vi "DGMM_PID_Trajectory tracking_0314.vi"() -> ()   [LabVIEW 2018]
doc: "Demonstrates the use of the Network Streams functions to send LED status to the myRIO target."
uses:
  <vilib>/addons/zeromq/socket_type.ctl
  <vilib>/ErrorRing/Error Ring.xnode
  <vilib>/vision/NI_Vision_Development_Module.lvlib
  <vilib>/addons/zeromq/zmq_context.lvclass
  <vilib>/addons/zeromq/zeromq.lvlib
  <vilib>/addons/zeromq/zmq_socket.lvclass
panel:
  in  "簇 11":T1={"next_state_x"=100000.0, "current_state_x"=1.0, "next_state_y"=100000.0, "current_state_y"=1.0}
  out "current_state_y":dbl
  out "current_state_x":dbl
  out "next_state_y":dbl
  out "next_state_x":dbl
  in  "簇 10":T2={"predicted_output_dr"=100000.0, "predicted_output_pr"=100000.0}
  in  "Operation":T3(ring)=enum."Erode"
  out "real_relative_point_y":dbl
  out "real_relative_point_x":dbl
  out "real_relative_start_point_y":dbl
  out "real_relative_start_point_x":dbl
  out "Bounding Box.Y Top 2":i32
  out "Bounding Box.X Left 2":i32
  out "Ki part":dbl
  out "Kd part":dbl
  out "Kp part":dbl
  out "Ki part":dbl
  out "Kd part":dbl
  out "Kp part":dbl
  in  "Ki":dbl=0.002
  in  "Kd":dbl=1e-05
  in  "Kp":dbl=0.005
  in  "Ki":dbl=0.002
  in  "Kd":dbl=1e-05
  in  "Kp":dbl=0.005
  out "添加的数组":dbl[](array[numeric])
  out "desired_relative_point_y":dbl=250.0
  out "desired_relative_point_x":dbl=200.0
  out "predicted_output_pr":dbl=20.0
  out "predicted_output_dr":dbl=8.0
  out "error_relative_point_y":dbl
  out "error_relative_point_x":dbl
  out "real_relative_end_point_y":dbl
  out "real_relative_end_point_x":dbl
  out "predicted_output_pr":dbl
  out "predicted_output_dr":dbl
  in  "打开仅尖端轨迹":bool
  out "仅尖端轨迹":T4(plugin-control)
  out "Bounding Box.Y Top":i32
  out "Bounding Box.X Left":i32
  out "curve_min_y":dbl
  out "curve_min_x":dbl
  out "curve_max_y":dbl
  out "curve_max_x":dbl
  out "relative_end_point_y":dbl
  out "relative_end_point_x":dbl
  out "delta_y":dbl
  out "delta_x":dbl
  out "pr":dbl
  out "tan(v)":dbl
  out "delta_velocity":dbl format="%#_10g"
  out "delta_time":dbl
  out "now time":timestamp[](array[timestamp])
  out "prev time":timestamp[](array[timestamp])
  out "delta_distance":dbl
  out "prev_end_point_y":dbl
  out "prev_end_point_x":dbl
  out "now_end_point_y":dbl
  out "now_end_point_x":dbl
  out "prev_end_point_y":dbl[](array[numeric])
  out "prev_end_point_x":dbl[](array[numeric])
  out "dr":dbl
  in  "Ar":sgl=11.0
  out "all parameters":dbl[][](array[numeric])
  out "direction angle":sgl[](array[numeric])
  out "dr":sgl
  out "strength":dbl[](array[numeric])
  out "场强":dbl
  out "end_point_y":T5
  out "end_point_x":dbl[](array[numeric])
  out "start_point_y":dbl[](array[numeric])
  out "start_point_x":dbl[](array[numeric])
  out "T":i32[](array[numeric])
  out "c":dbl[](array[numeric])
  out "b":dbl[](array[numeric])
  out "a\na":dbl[](array[numeric])
  out "c":dbl
  out "b":dbl
  out "a":dbl
  out "Angles (deg)":sgl[](array[numeric]) format="%.2f"
  in  "wr":sgl
  in  "打开轨迹":bool
  out "中心轨迹和尖端轨迹":T4(plugin-control)
  out "end_y":dbl
  out "end_x":dbl
  out "start_y":dbl
  out "start_x":dbl
  out "Image Pixels (U8)":u8[][](array[numeric])
  in  "Poly":dbl
  out "中心轨迹":T4(plugin-control)
  in  "保存按钮":bool
  out "Object Center":cluster{"X":sgl, "Y":sgl}
  out "黑白图":T4(plugin-control)
  in  "Number of Erosion":i32=5
  in  "Settings":T6={"Objects"=1, "Threshold"=128, "Reject Border"=FALSE, "Fill Holes"=FALSE, "Min Object Size"=TRUE, "Min Size"=3000, "Max Object Size"=FALSE, "Max Size"=100, "Show Search Area"=TRUE, "Show Center"=TRUE, "Show Bounding Box"=TRUE} {"Objects" items=["Bright Objects", "Dark Objects"]; "Threshold" min=1 max=999999999 step=1; "Max Size" min=1 max=999999999 step=1; "Min Size" min=1 max=999999999 step=1}
  out "Objects":T7(array[cluster]) {"Aspect Ratio" format="%.2f"; "Orientation" format="%.2f"; "Area" format="%.2f"; "Object Center"."Y" format="%.2f"; "Object Center"."X" format="%.2f"}
  in  "Search Rect (entire image)":T8={"Left"=160, "Top"=740, "Right"=1900, "Bottom"=1620, "Rotation"=0.0} {"Rotation" format="%.2f"; "Left" scale=0.0..1024.0; "Right" scale=0.0..1024.0}
  in  "Range":cluster{"Lower value":sgl, "Upper value":sgl}={"Lower value"=181.0, "Upper value"=255.0} {"Upper value" format="%.2f"; "Lower value" format="%.2f"}
  out "原图":T4(plugin-control)
  in  "停止":bool
  out "T":i32
  out "T":i32
  in  "磁场变换":bool=TRUE
  in  "Pause":bool
  out "Array":ext[](array[numeric])
  in  "Parameter Settings":T9(tab)=enum."Rotating Field" caption="Field Types"
  in  "Ag":dbl
  in  "dg":dbl
  in  "pg":dbl
  in  "fg":dbl
  in  "AoOF":dbl
  in  "fo":sgl
  in  "do":sgl
  in  "oo":sgl
  in  "po":sgl
  in  "cc":sgl
  in  "pc":sgl
  in  "wc":sgl
  in  "dc":sgl
  in  "Ac":dbl
  in  "Dis phase step":dbl
  in  "Dis phase frequency (Hz)":dbl
  in  "Dis tumbling frequency (Hz)":dbl
  in  "Dis strength(mT)":dbl
  in  "Swa strength (mT)":dbl
  in  "Swa frequency (Hz)":dbl
  in  "Swa pitch angle (deg)":dbl
  in  "Swa direction angle (deg)":dbl
  in  "Swa ratio":dbl=1.0
  in  "Pitch Angle (rotating around Constant, deg)":dbl
  in  "Ratio (A/C)":sgl
  in  "Direction Angle (deg)":sgl
  in  "Pitch Angle (rotating around Origin, deg)":sgl
  in  "Frequency (Hz)":sgl
  in  "Strength (mT)":dbl
  in  "Ar 2":dbl caption="Ar"
  in  "ratio":sgl
  in  "pr  2":sgl
  in  "dr  2":sgl
  in  "wr  2":sgl
  in  "p_x":sgl
  out "Numeric 5":i32
  in  "Stop":bool
  out "error out":errorcluster
  in  "Target IP Address":string="172.22.11.2"
  # "Overview: Magnetic field calculation, and send parameters to myRIO\nInstructions:\n1. Verify the value of Target IP Address. Set Visa resource name.\n2. Ensure RT Main.vi is already running. \n3. Run this VI. Set parameters of magnetic field."
  # "Strength (mT)"
  # "Frequency (Hz)"
  # "Pitch Angle (deg)"
  # "Direction Angle (deg)"
  # "Strength (mT)"
  # "Pitch Angle (deg)"
  # "Direction Angle (deg)"
  # "Frequency (Hz)"
  # "Strength (mT)"
  # "Oscilation Frequency (Hz)"
  # "Oscilation Angle (deg)"
  # "Pitch Angle (deg)"
  # "Direction Angle (deg)"
  # "Strength (mT)"
  # "Frequency (Hz)"
  # "Pitch Angle (deg)"
  # "Direction Angle (deg)"
  # "Conical Angle (deg)"
  # "Strength (mT)"
  # "Tumbling Frequency (Hz)"
  # "Phase Frequency (Hz)"
  # "Phase Step"
  # "Strength (mT)"
  # "Frequency (Hz)"
  # "Pitch Angle (deg)"
  # "Direction Angle (deg)"
  # "Ratio"
  # "Strength (mT)"
  # "Frequency (Hz)"
  # "Ratio (A/C)"
  # "Direction Angle (deg)"
  # "Pitch Angle (rotating around Origin, deg)"
  # "Pitch Angle (rotating around Constant, deg)"
  # "Strength (mT)"
  # "Frequency (Hz)"
  # "Pitch Angle Y (deg)"
  # "Pitch Angle X (deg)"
  # "Direction Angle (deg)"
  # "ratio (l/s)"
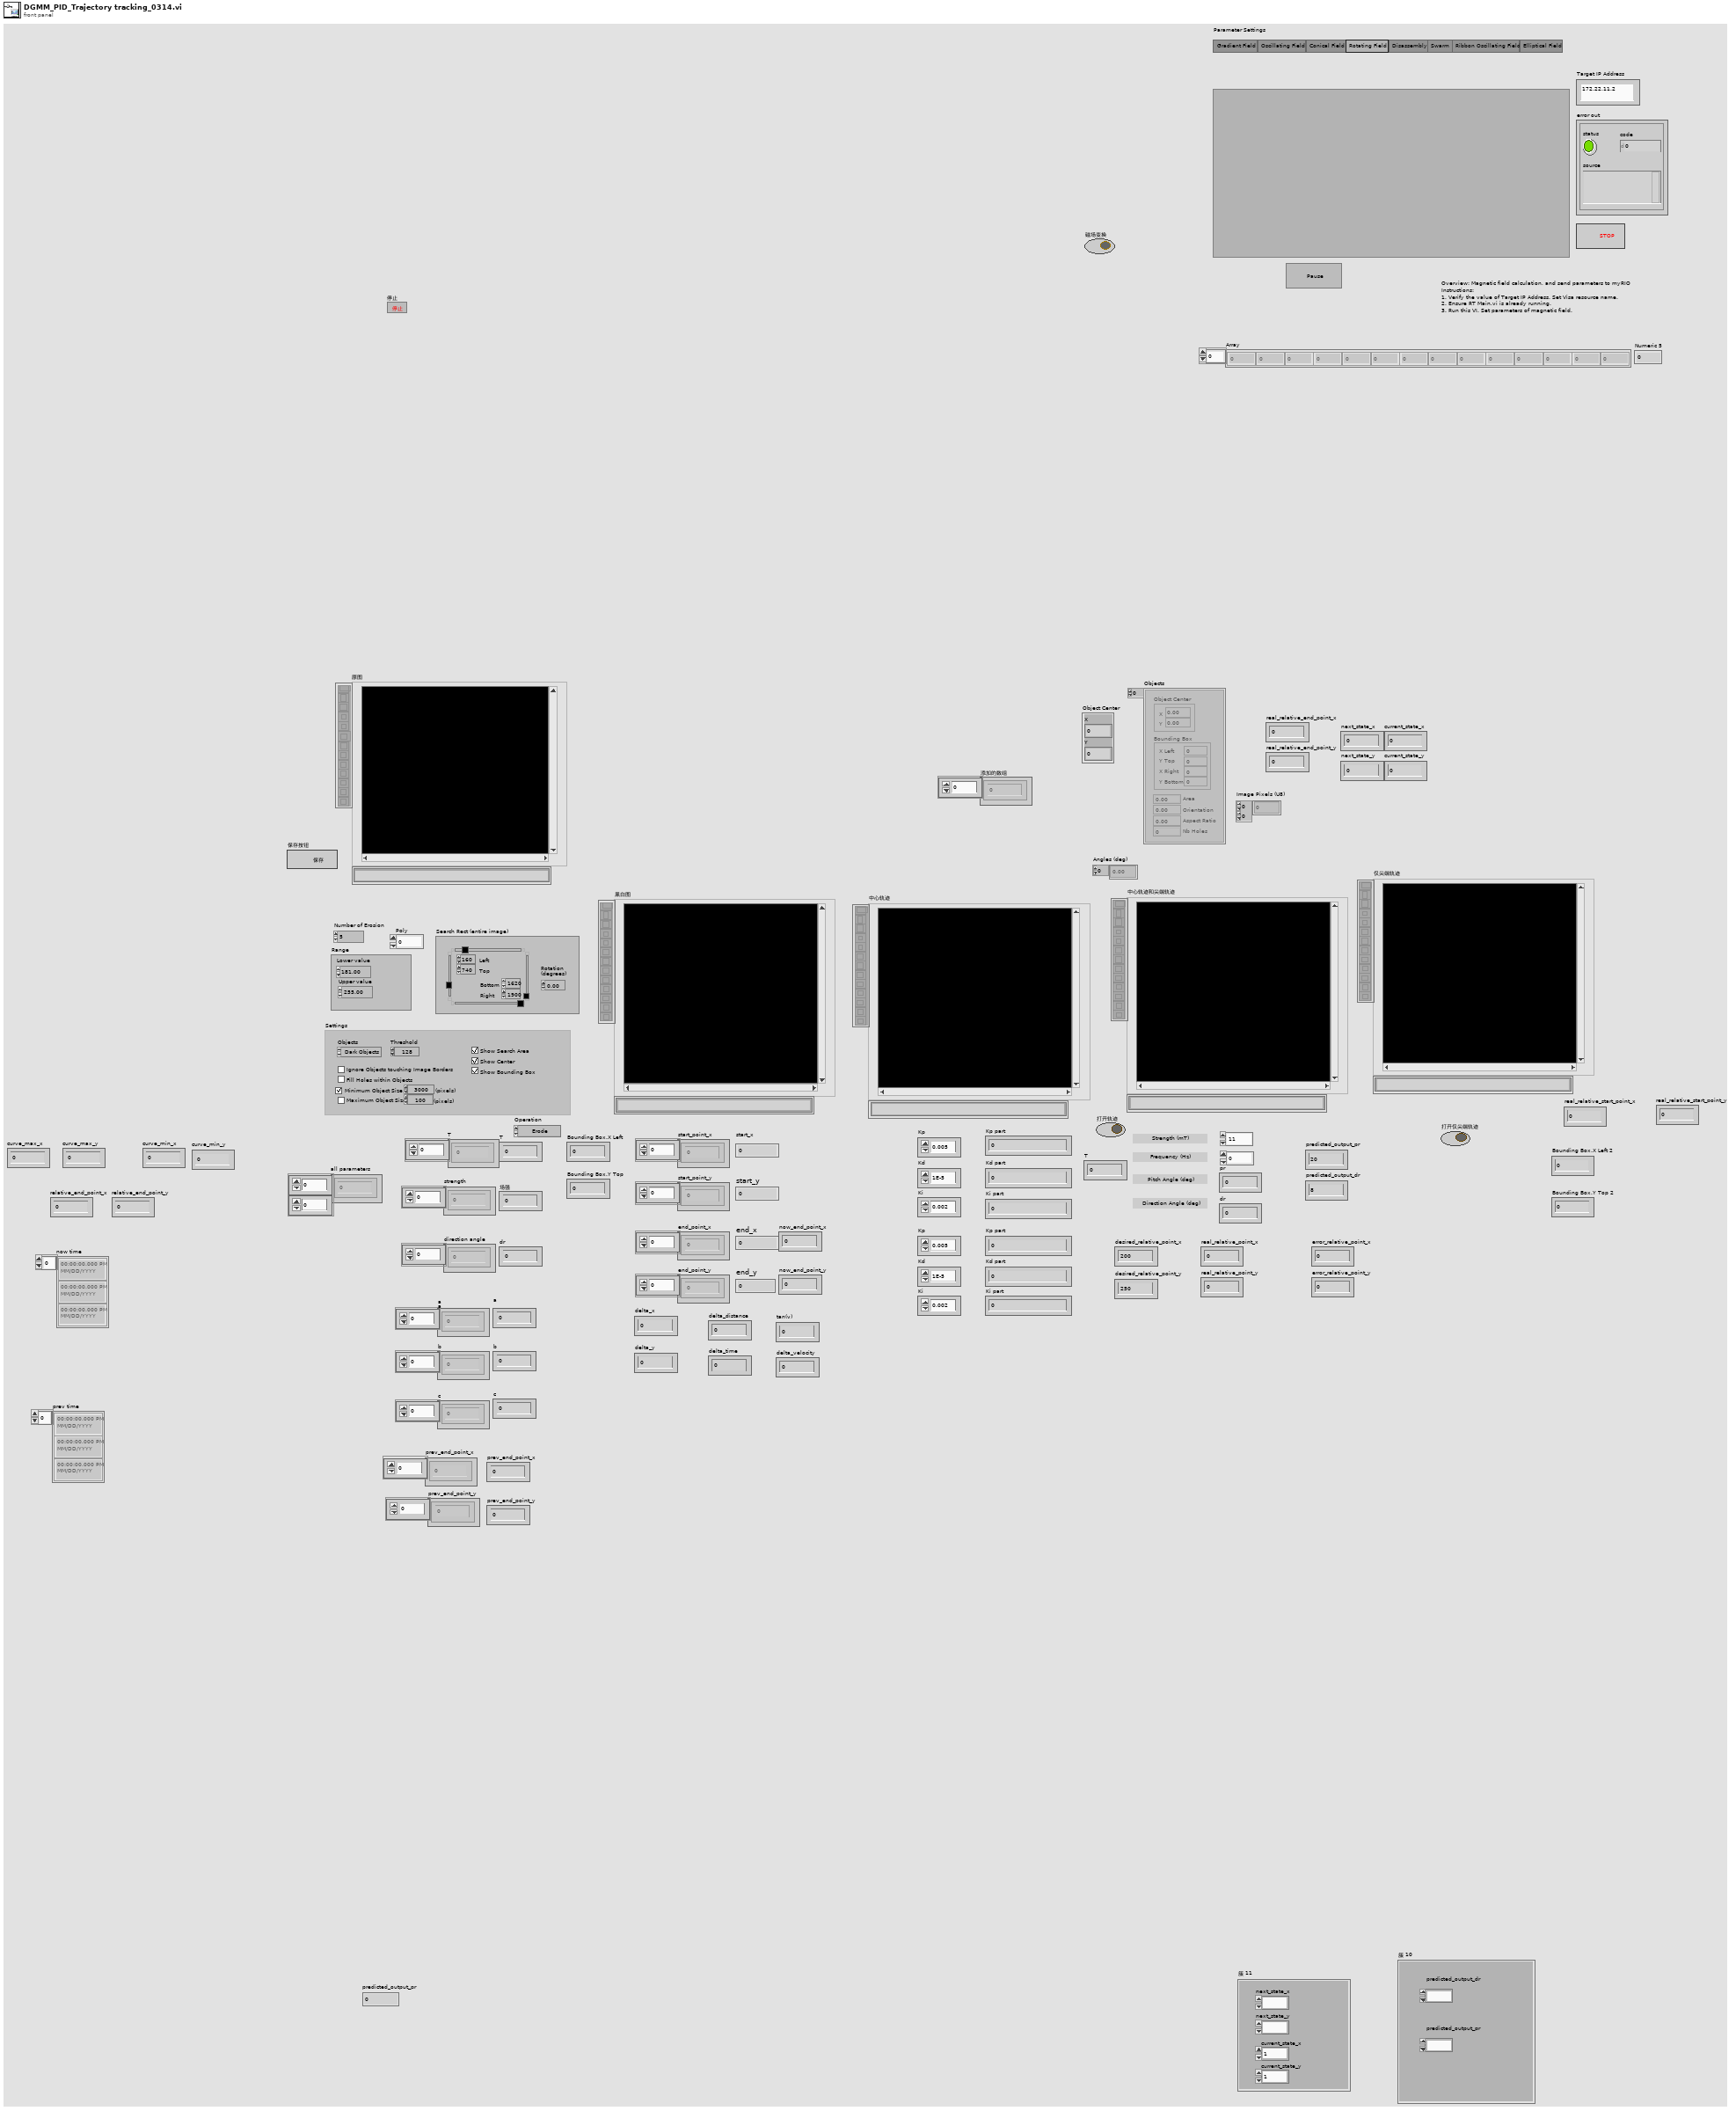
[diagram p1: front panel]
types:
  T1 = cluster{"next_state_x":ext, "current_state_x":dbl, "next_state_y":ext, "current_state_y":dbl}
  T2 = cluster{"predicted_output_dr":ext, "predicted_output_pr":ext}
  T3 = enum32{"AutoM", "Close", "Dilate", "Erode", "Gradient", "Gradient in", "Gradient out", "HitMiss", "Open", "PClose", "POpen", "Thick", "Thin"}
  T4 = typedef "IMAQ Image.ctl" = refnum<image>
  T5 = typedef "控件 3.ctl" = dbl[]
  T6 = cluster{"Objects":u16, "Threshold":i32, "Reject Border":bool, "Fill Holes":bool, "Min Object Size":bool, "Min Size":i32, "Max Object Size":bool, "Max Size":i32, "Show Search Area":bool, "Show Center":bool, "Show Bounding Box":bool}
  T7 = cluster{"Object Center":cluster{"X":sgl, "Y":sgl}, "Bounding Box":cluster{"X Left":i32, "Y Top":i32, "X Right":i32, "Y Bottom":i32}, "Area":sgl, "Orientation":sgl, "Aspect Ratio":sgl, "Nb Holes":i32}[]
  T8 = typedef "IMAQ Rectangle" = cluster{"Left":i32, "Top":i32, "Right":i32, "Bottom":i32, "Rotation":dbl}
  T9 = enum32{"Gradient Field ", "Oscillating Field", "Conical Field", "Rotating Field", "Disassembly", "Swarm", "Ribbon Oscillating Field", "Elliptical Field"}
  T10 = typedef "zeromq.lvlib/socket_type.ctl" = enum8{"ZMQ_PAIR", "ZMQ_PUB", "ZMQ_SUB", "ZMQ_REQ", "ZMQ_REP", "ZMQ_DEALER", "ZMQ_ROUTER", "ZMQ_PULL", "ZMQ_PUSH", "ZMQ_XPUB", "ZMQ_XSUB", "ZMQ_STREAM", "ZMQ_SERVER", "ZMQ_CLIENT", "ZMQ_RADIO", "ZMQ_DISH", "ZMQ_GATHER", "ZMQ_SCATTER", "ZMQ_DGRAM"}
  T11 = typedef "Image Type" = u32
  T12 = cluster{"Object Center":cluster{"X":sgl, "Y":sgl}, "Bounding Box":cluster{"X Left":i32, "Y Top":i32, "X Right":i32, "Y Bottom":i32}, "Area":sgl, "Orientation":sgl, "Aspect Ratio":sgl, "Nb Holes":i32}
  T13 = cluster{"X Left":i32, "Y Top":i32, "X Right":i32, "Y Bottom":i32, "Rotation":dbl}
  T14 = typedef "ROI Descriptor" = cluster{"Global Rectangle":i32[], "Contours":cluster{"ID":enum32{"External", "Internal"}, "Type":u32, "Coordinates":i32[]}[]}
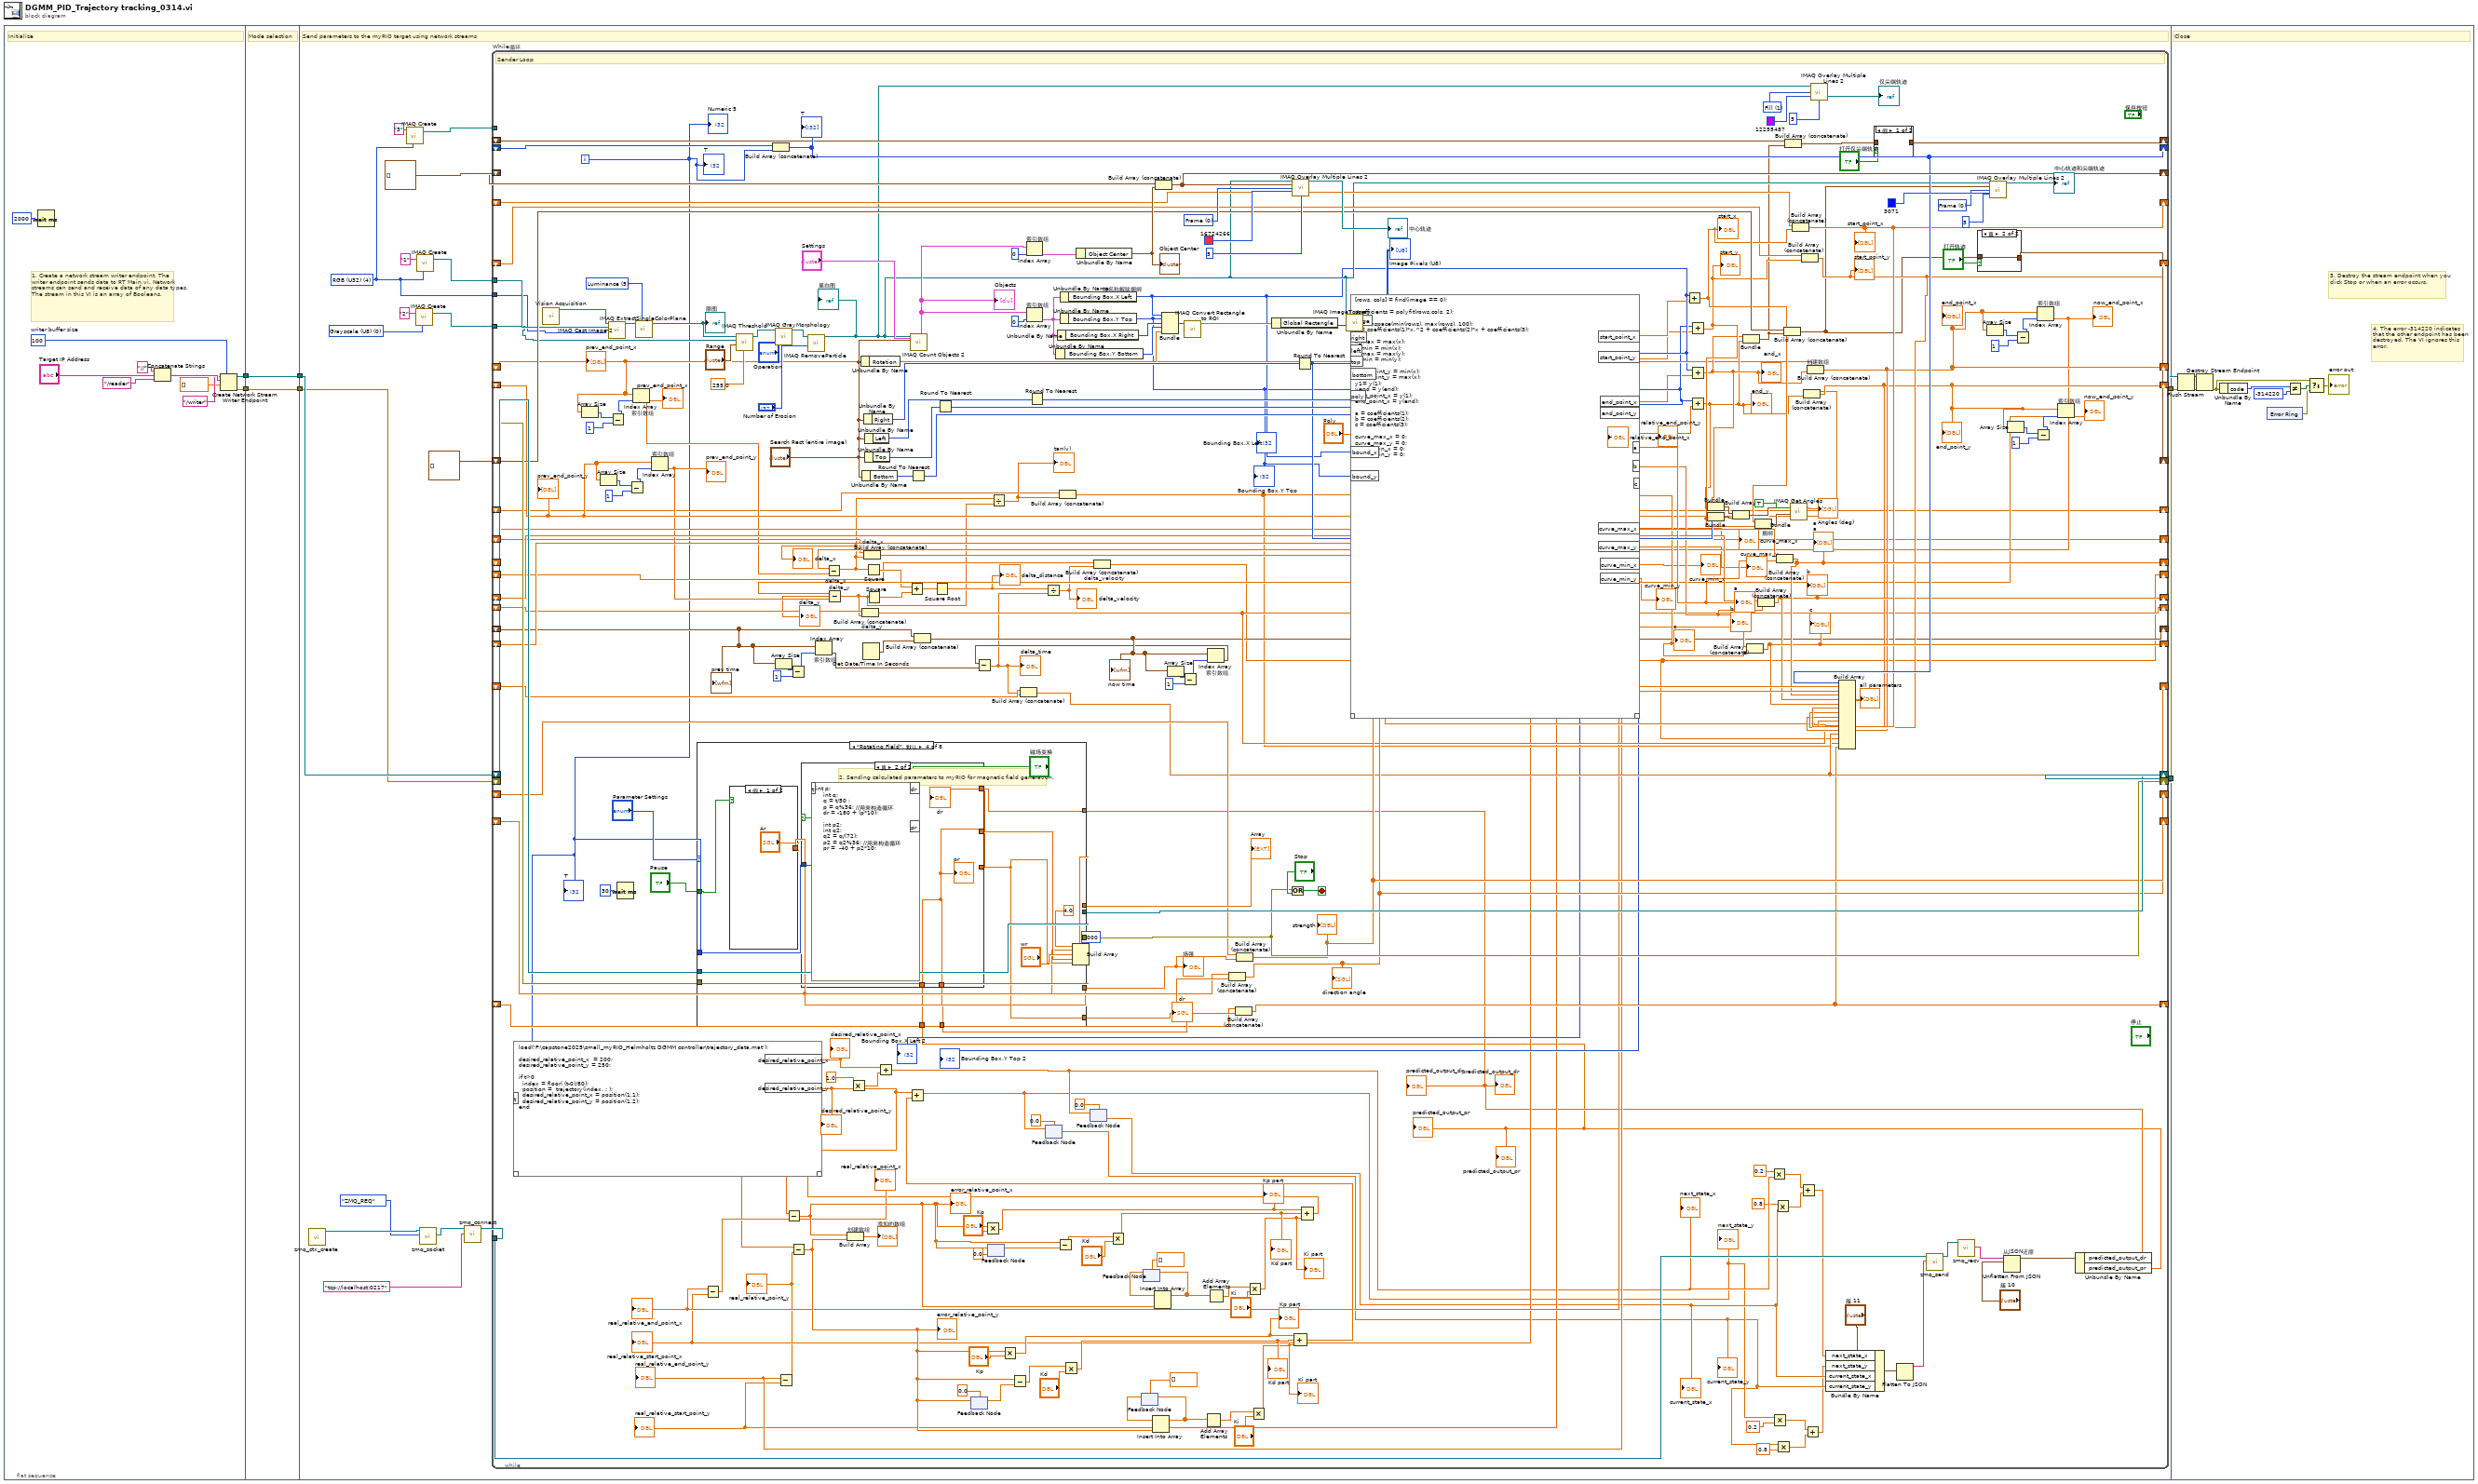
[diagram p0: block diagram]
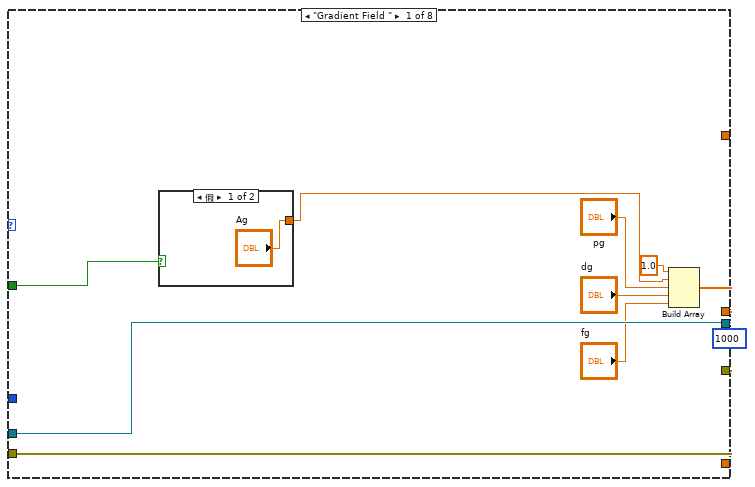
[diagram p4: hidden frame]
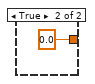
[diagram p5: hidden frame]
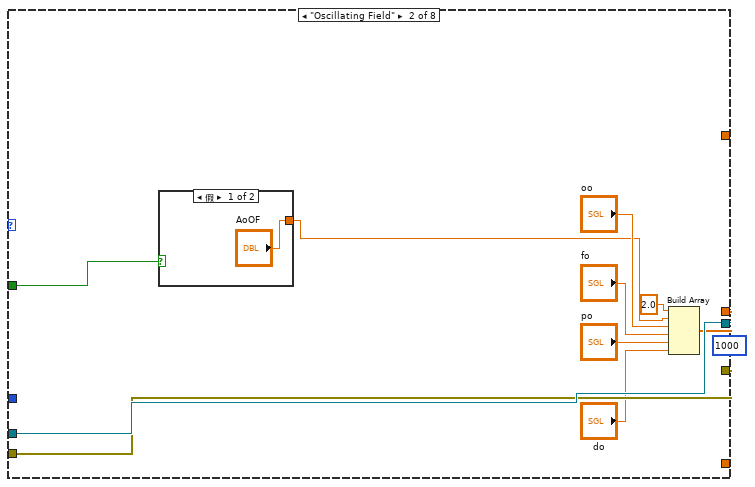
[diagram p6: hidden frame]
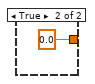
[diagram p7: hidden frame]
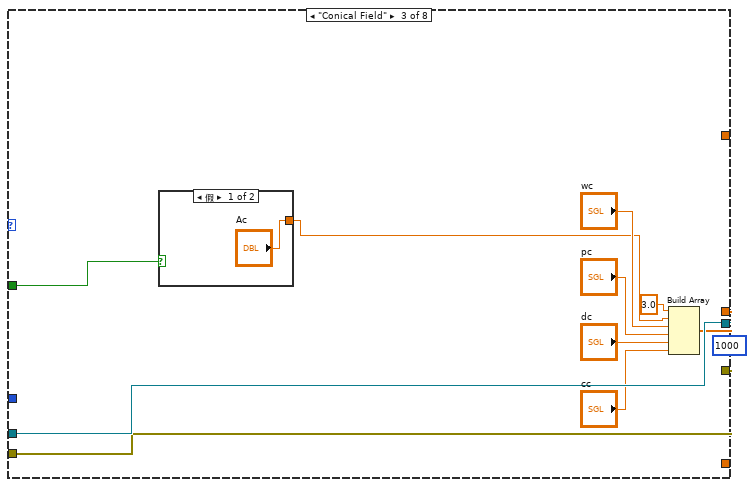
[diagram p8: hidden frame]
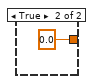
[diagram p9: hidden frame]
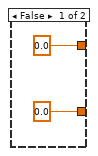
[diagram p10: hidden frame]
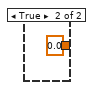
[diagram p11: hidden frame]
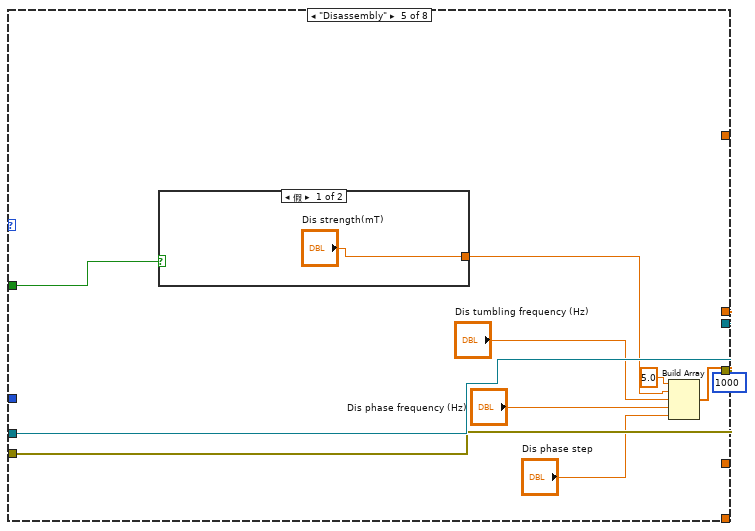
[diagram p12: hidden frame]
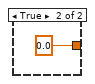
[diagram p13: hidden frame]
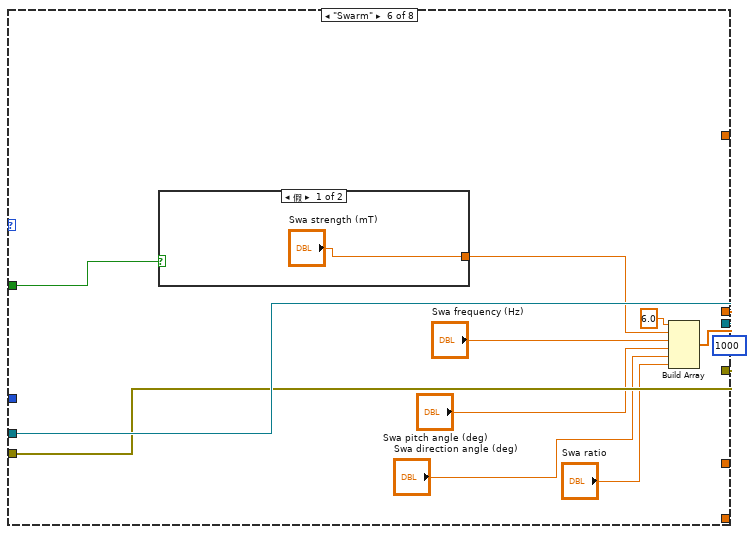
[diagram p14: hidden frame]
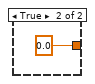
[diagram p15: hidden frame]
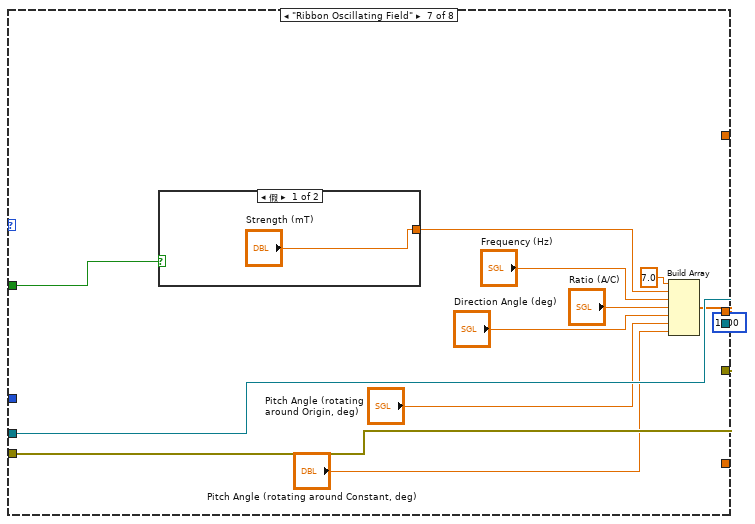
[diagram p16: hidden frame]
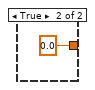
[diagram p17: hidden frame]
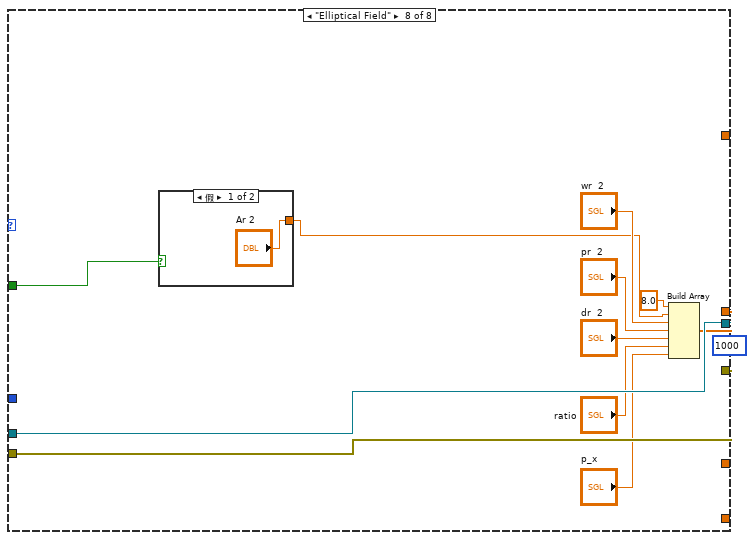
[diagram p18: hidden frame]
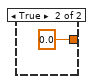
[diagram p19: hidden frame]
diagram:
  n1 = flat-sequence {
    tunnel: [w11] -> w2
    tunnel: [w10] -> w1
    tunnel: [w18] -> w4
    tunnel: [w17] -> w3
    tunnel: w1 -> [w17]
    tunnel: w2 -> [w18]
    tunnel: [w35] -> w6
    tunnel: w4 -> [w37]
    tunnel: [w34] -> w5
    tunnel: w3 -> [w36]
    tunnel: w6 -> [w408]
    tunnel: w5 -> [w405]
    frame #0 {
      w9 = 100  # writer buffer size
      # "1. Create a network stream writer endpoint. The writer endpoint sends data to RT Main.vi. Network streams can send and receive data of any data types. The stream in this VI is an array of Booleans."
      # "Initialize"
      n2 = Wait (ms)(milliseconds to wait=2000) -> ()  [unwired: 1 out]
      n3 = Concatenate Strings("//", "Target IP Address", "/reader") -> (w16:string)
      n4 = Create Network Stream Writer Endpoint(7:w9, 9:dbl[] [], 10:w16, 11:"/writer" ("reader name")) -> (0:w10:errorcluster, 3:w11:refnum<k21>)  [unwired: 3 in]
    }
    frame #1 {
      # "Mode selection"
    }
    frame #2 {
      w31 = T11 0 items=["Grayscale (U8)", "Grayscale (I16)", "Grayscale (SGL)", "Complex (CSG)", "RGB (U32)", "HSL (U32)", "RGB (U64)", "Grayscale (U16)"] ("Image Type")
      w24 = T11 4 items=["Grayscale (U8)", "Grayscale (I16)", "Grayscale (SGL)", "Complex (CSG)", "RGB (U32)", "HSL (U32)", "RGB (U64)", "Grayscale (U16)"] ("Image Type")
      # "Send parameters to the myRIO target using network streams"
      n5 = call <vilib>:"zmq_ctx_create.vi"() -> ("context out"=w22:refnum<class "zmq_context.lvclass">)  [unwired: 4 in, 1 out]
      n6 = call "IMAQ Create"("Image Name"="3", "Image Type"=w24) -> ("New Image"=w27:T4)  [unwired: 3 in, 1 out]
      n7 = call "IMAQ Create"("Image Name"="2", "Image Type"=w31) -> ("New Image"=w29:T4)  [unwired: 3 in, 1 out]
      n8 = call "IMAQ Create"("Image Name"="1", "Image Type"=w24) -> ("New Image"=w30:T4)  [unwired: 3 in, 1 out]
      n9 = call <vilib>:"zmq_socket.vi"("socket type"=socket_type."ZMQ_REQ", "context in"=w22) -> ("socket out"=w23:refnum<class "zmq_socket.lvclass">)  [unwired: 3 in, 2 out]
      n10 = call <vilib>:"zmq_connect.vi"("endpoint"="tcp://localhost:0217", "socket in"=w23) -> ("socket out"=w19:refnum<class "zmq_socket.lvclass">)  [unwired: 2 in, 1 out]
      n11 = while "While循环" {
        shift-right: [w263] -> w34
        shift-left: w36 -> [w265]
        shift-right: [w264] -> w35
        shift-left: w37 -> [w266]
        tunnel: w30 -> [w217]
        tunnel: w29 -> [w216]
        tunnel: w27 -> [_]
        shift-right: [w213] -> _
        shift-left: cluster{"X":dbl, "Y":dbl}[] [] -> [w218]
        shift-right: [w219] -> _
        shift-left: cluster{"X":dbl, "Y":dbl}[] [] -> [w220]
        tunnel: w24 -> [w215]
        shift-right: [w185] -> _
        shift-left: _ -> [w205]
        shift-right: [w180] -> _
        shift-left: _ -> [w203]
        shift-right: [w184] -> _
        shift-left: _ -> [w200]
        shift-right: [w188] -> _
        shift-left: _ -> [w199]
        shift-right: [w183] -> _
        shift-left: _ -> [w197]
        shift-right: [w182] -> _
        shift-left: _ -> [w195]
        shift-right: [w176] -> _
        shift-left: _ -> [w168]
        shift-right: [w172] -> _
        shift-left: _ -> [w164]
        shift-right: [w187] -> _
        shift-left: _ -> [w191]
        shift-right: [w186] -> _
        shift-left: _ -> [w189]
        shift-right: [w153] -> _
        shift-left: _ -> [w155]
        shift-right: [w152] -> _
        shift-left: _ -> [w154]
        shift-right: [w142] -> _
        shift-left: _ -> [w147]
        shift-right: [w139] -> _
        shift-left: _ -> [w140]
        shift-right: [w135] -> _
        shift-left: _ -> [w136]
        shift-right: [w130] -> _
        shift-left: _ -> [w131]
        shift-right: [w122] -> _
        shift-left: _ -> [w123]
        shift-right: [w116] -> _
        shift-left: _ -> [w117]
        tunnel: w19 -> [w56]
        i -> [w110]
        stop <- w259 stop-if-true
        w118 = u32 1 items=["Frame", "Fill"] ("Drawing Mode (Frame)")
        w125 = u32 0 items=["Frame", "Fill"] ("Drawing Mode (Frame)")
        w246 = u32 0 items=["Frame", "Fill"] ("Drawing Mode (Frame)")
        w256 = 5 items=["Red", "Green", "Blue", "Hue", "Saturation", "Luminance", "Value", "Intensity"] ("Color Plane")
        # "2. Sending calculated parameters to myRIO for magnetic field generation."
        # "Sender Loop"
        n12 = script code="load('F:\\capstone2025\\small_myRIO_Helmholtz DGMM controller\\trajectory_data.mat');\n\ndesired_relative_point_x  = 200;\ndesired_relative_point_y = 250;\n\nif t>0\n  index = floor( (t-0)/80); \n  position =  trajectory(index, : );\n  desired_relative_point_x = position(1,1);\n  desired_relative_point_y = position(1,2);\nend"("t"=w110) -> ("desired_relative_point_x"=w64:dbl, "desired_relative_point_y"=w65:dbl)  [unwired: 1 in, 1 out]
        "desired_relative_point_x" <- w64
        "desired_relative_point_y" <- w65
        n13 = call "Vision Acquisition"() -> ("Image Out"=w244:T4)  [unwired: 23 in, 4 out]
        n14 = Array Size(array=w168) -> (size(s)=w170:i32)
        n15 = Array Size(array=w164) -> (size(s)=w166:i32)
        n16 = call "IMAQ Cast Image 2"("Image Src"=w244, "Image Dst"=w217, "Image Type"=w215) -> ("Image Dst Out"=w257:T4)  [unwired: 11 in, 1 out]
        n17 = Subtract(x=w170, y=1) -> (x-y=w169:i32)
        n18 = Wait (ms)(milliseconds to wait=u32 30 ("等待时间（毫秒）")) -> ()  [unwired: 1 out]
        n19 = Subtract(x=w166, y=1) -> (x-y=w165:i32)
        n20 = Index Array "索引数组"(array=w168, index=w169) -> (element=w162:dbl)
        "prev_end_point_x" <- w162
        n21 = call "IMAQ ExtractSingleColorPlane"("Color Plane"=w256, "Image Src"=w257) -> ("Image Dst Out"=w255:T4)  [unwired: 8 in, 1 out]
        "原图" <- w255
        n22 = Index Array "索引数组"(array=w164, index=w165) -> (element=w161:dbl)
        "prev_end_point_y" <- w161
        n23 = call "IMAQ Threshold"("Replace Value"=sgl 255.0, "Range"="Range", "Image Dst"=w216, "Image Src"=w255) -> ("Image Dst Out"=w71:T4)  [unwired: 6 in, 1 out]
        n24 = Build Array (concatenate)(w199, w110) -> (w188:i32[])
        "T" <- w188
        n25 = call "IMAQ GrayMorphology"("Operation"="Operation", "Image Src"=w71) -> ("Image Dst Out"=w70:T4)  [unwired: 8 in, 1 out]
        n26 = Array Size(array=w147) -> (size(s)=w150:i32)
        n27 = Subtract(x=w150, y=1) -> (x-y=w149:i32)
        n28 = call "IMAQ RemoveParticle"("Number of Erosion"="Number of Erosion", "Image Src"=w70) -> ("Image Dst Out"=w114:T4)  [unwired: 8 in, 1 out]
        "黑白图" <- w114
        n29 = Index Array "索引数组"(array=w147, index=w149) -> (element=w146:timestamp)
        n30 = Unbundle By Name("Search Rect (entire image)") -> ("Rotation"=w241:dbl)
        n31 = Unbundle By Name("Search Rect (entire image)") -> ("Bottom"=w225:i32)
        n32 = Get Date/Time In Seconds() -> (seconds since 1Jan1904=w151:timestamp)
        n33 = Unbundle By Name("Search Rect (entire image)") -> ("Right"=w229:i32)
        n34 = Unbundle By Name("Search Rect (entire image)") -> ("Left"=w228:i32)
        n35 = Unbundle By Name("Search Rect (entire image)") -> ("Top"=w227:i32)
        n36 = Round To Nearest(number=w225) -> (nearest integer value=w224:i32)
        n37 = call "IMAQ Count Objects 2"("Settings"="Settings", "Search Rect (entire image)"="Search Rect (entire image)", "Image"=w114) -> ("Objects"=w243:T7)  [unwired: 4 in, 4 out]
        "Objects" <- w243
        n38 = Build Array (concatenate)(w147, w151) -> (w142:timestamp[])
        "now time" <- w142
        n39 = Round To Nearest(number=w227) -> (nearest integer value=w226:i32)
        n40 = feedback #1(0.0) -> (w92:dbl)
        n41 = feedback #2(0.0) -> (w106:dbl)
        n42 = Index Array "索引数组"(array=w243, index=0 ("索引")) -> (element=w249:T12)
        n43 = Index Array "索引数组"(array=w243, index=0 ("索引")) -> (element=w239:T12)
        n44 = Round To Nearest(number=w228) -> (nearest integer value=w222:i32)
        n45 = feedback #3(0.0) -> (w42:dbl)
        "current_state_y" <- w42
        n46 = Unbundle By Name(w239) -> ("Bounding Box.Y Bottom"=w233:i32)
        n47 = Unbundle By Name(w239) -> ("Bounding Box.X Right"=w234:i32)
        n48 = Unbundle By Name "按名称解除捆绑"(w239) -> ("Bounding Box.X Left"=w79:i32)
        "Bounding Box.X Left" <- w79
        "Bounding Box.X Left 2" <- w79
        n49 = Unbundle By Name(w239) -> ("Bounding Box.Y Top"=w78:i32)
        "Bounding Box.Y Top" <- w78
        "Bounding Box.Y Top 2" <- w78
        n50 = Unbundle By Name(w249) -> ("Object Center"=w248:cluster{"X":sgl, "Y":sgl})
        "Object Center" <- w248
        n51 = feedback #4(0.0) -> (w49:dbl)
        "current_state_x" <- w49
        n52 = feedback #5(dbl[] []) -> (w87:dbl[])
        n53 = feedback #6(dbl[] []) -> (w101:dbl[])
        n54 = Build Array (concatenate)(w220, w248) -> (w219:cluster{"X":dbl, "Y":dbl}[])
        n55 = Bundle("X Left"=w79, "Y Top"=w78, "X Right"=w234, "Y Bottom"=w233, "Rotation"=w241) -> (w240:T13)  [unwired: 1 in]
        n56 = Array Size(array=w142) -> (size(s)=w145:i32)
        n57 = Subtract(x=w145, y=1) -> (x-y=w144:i32)
        n58 = call "IMAQ Convert Rectangle to ROI"("Rectangle"=w240) -> ("ROI Descriptor"=w238:T14)  [unwired: 8 in, 1 out]
        n59 = Index Array "索引数组"(array=w142, index=w144) -> (element=w141:timestamp)
        n60 = Subtract(x=w141, y=w146) -> (x-y=w138:dbl)
        "delta_time" <- w138
        n61 = Build Array (concatenate)(w140, w138) -> (w139:dbl[])
        n62 = Unbundle By Name(w238) -> ("Global Rectangle"=w223:i32[])
        n63 = call "IMAQ Overlay Multiple Lines 2"("Image"=w114, "Line End Points"=w219, "Drawing Mode (Frame)"=w246, "Color"=u32 16724266, "Width"=u32 5) -> ("Image Out"=→"中心轨迹":T4)  [unwired: 9 in, 1 out]
        n64 = Round To Nearest(number=w229) -> (nearest integer value=w206:i32)
        n65 = call "IMAQ ImageToArray"("Optional Rectangle"=w223, "Image"=w114) -> ("Image Pixels (U8)"=w235:u8[][])  [unwired: 2 in, 4 out]
        "Image Pixels (U8)" <- w235
        n66 = script code="[rows, cols] = find(image == 0); \n\ncoefficients = polyfit(rows,cols, 2);\n\nx = linspace(min(rows), max(rows), 100); \ny = coefficients(1)*x.^2 + coefficients(2)*x + coefficients(3);\n\nx_max = max(x);\nx_min = min(x);\ny_max = max(y);\ny_min = min(y);\n\nstart_point_y = min(x);\nend_point_y = max(x);\ny1= y(1);\nyend = y(end);\nstart_point_x = y(1);\nend_point_x = y(end);\n\na = coefficients(1);\nb = coefficients(2);\nc = coefficients(3);\n\ncurve_max_x = 0;\ncurve_max_y = 0;\ncurve_min_x = 0;\ncurve_min_y = 0;"("image"=w235, "poly"="Poly", "right"=w206, "left"=w222, "top"=w226, "bottom"=w224, "bound_x"=w79, "bound_y"=w78) -> ("start_point_x"=w76:dbl, "start_point_y"=w73:dbl, "end_point_x"=w77:dbl, "end_point_y"=w74:dbl, "a"=w204:dbl, "b"=w202:dbl, "c"=w201:dbl, "curve_max_x"=→"curve_max_x":dbl, "curve_max_y"=→"curve_max_y":dbl, "curve_min_x"=→"curve_min_x":dbl, "curve_min_y"=→"curve_min_y":dbl)  [unwired: 1 in, 1 out]
        "a" <- w204
        "b" <- w202
        "c" <- w201
        "relative_end_point_x" <- w77
        "relative_end_point_y" <- w74
        "real_relative_end_point_x" <- w77
        "real_relative_end_point_y" <- w74
        "real_relative_start_point_x" <- w76
        "real_relative_start_point_y" <- w73
        n67 = Subtract(x=w77, y=w76) -> (x-y=w75:dbl)
        "real_relative_point_x" <- w75
        n68 = Subtract(x=w74, y=w73) -> (x-y=w72:dbl)
        "real_relative_point_y" <- w72
        n69 = Subtract(x=w64, y=w75) -> (x-y=w100:dbl)
        "error_relative_point_x" <- w100
        n70 = Subtract(x=w65, y=w72) -> (x-y=w85:dbl)
        "error_relative_point_y" <- w85
        n71 = Build Array "创建数组"(w100, w85) -> (→"添加的数组":dbl[])
        n72 = feedback-in #1(w85) -> ()
        n73 = Multiply(x=w100, y="Kp") -> (x*y=w107:dbl)
        "Kp part" <- w107
        n74 = feedback-in #2(w100) -> ()
        n75 = Multiply(x=w85, y="Kp") -> (x*y=w93:dbl)
        "Kp part" <- w93
        n76 = Subtract(x=w85, y=w92) -> (x-y=w90:dbl)
        n77 = Subtract(x=w100, y=w106) -> (x-y=w104:dbl)
        n78 = Multiply(x=w90, y="Kd") -> (x*y=w88:dbl)
        "Kd part" <- w88
        n79 = Multiply(x=w104, y="Kd") -> (x*y=w102:dbl)
        "Kd part" <- w102
        n80 = Insert Into Array(array=w87, new element=w85) -> (w86:dbl[])  [unwired: 1 in]
        n81 = feedback-in #5(w86) -> ()
        n82 = Insert Into Array(array=w101, new element=w100) -> (w99:dbl[])  [unwired: 1 in]
        n83 = feedback-in #6(w99) -> ()
        n84 = Add Array Elements(numeric array=w86) -> (sum=w83:dbl)
        n85 = Add Array Elements(numeric array=w99) -> (sum=w97:dbl)
        n86 = Multiply(x=w97, y="Ki") -> (x*y=w95:dbl)
        "Ki part" <- w95
        n87 = Multiply(x=w83, y="Ki") -> (x*y=w81:dbl)
        "Ki part" <- w81
        n88 = Compound Arithmetic op=ADD(w93, w88, w81) -> (w80:dbl)
        n89 = Add(x=w65, y=w80) -> (x+y=w44:dbl)
        "next_state_y" <- w44
        n90 = feedback-in #3(w44) -> ()
        n91 = Compound Arithmetic op=ADD(w107, w102, w95) -> (w68:dbl)
        n92 = Multiply(x=1.0, y=w68) -> (x*y=w66:dbl)
        n93 = Add(x=w64, y=w66) -> (x+y=w51:dbl)
        "next_state_x" <- w51
        n94 = feedback-in #4(w51) -> ()
        n95 = Add(x=w79, y=w76) -> (x+y=w198:dbl)
        "start_x" <- w198
        n96 = Add(x=w78, y=w73) -> (x+y=w196:dbl)
        "start_y" <- w196
        n97 = Add(x=w79, y=w77) -> (x+y=w194:dbl)
        "end_x" <- w194
        n98 = Add(x=w78, y=w74) -> (x+y=w193:dbl)
        "end_y" <- w193
        n99 = Bundle(w194, w193) -> (w210:cluster{dbl, dbl})  [unwired: 1 in]
        n100 = Bundle(w206, w196) -> (w209:cluster{i32, dbl})  [unwired: 1 in]
        n101 = Build Array(w210, w209) -> (w208:cluster{dbl, dbl}[])
        n102 = Bundle(w194, w193) -> (w112:cluster{dbl, dbl})  [unwired: 1 in]
        n103 = Build Array (concatenate)(w200, w201) -> (w184:dbl[])
        "c" <- w184
        n104 = Bundle "捆绑"(w198, w196) -> (w211:cluster{dbl, dbl})  [unwired: 1 in]
        n105 = Build Array (concatenate)(w203, w202) -> (w180:dbl[])
        "b" <- w180
        n106 = Multiply(x=0.2, y=w51) -> (x*y=w47:dbl)
        n107 = Multiply(x=w44, y=0.2 ("x+y")) -> (x*y=w40:dbl)
        n108 = Multiply(x=0.8, y=w49) -> (x*y=w46:dbl)
        n109 = Multiply(x=w42, y=0.8) -> (x*y=w39:dbl)
        n110 = Build Array (concatenate)(w205, w204) -> (w185:dbl[])
        "a\na" <- w185
        n111 = Build Array (concatenate)(w218, w112) -> (w113:cluster{"X":dbl, "Y":dbl}[])
        n112 = Build Array (concatenate)(w117, w112) -> (w111:cluster{dbl, dbl}[])
        n113 = call "IMAQ Get Angles"("Vertex"=w211, "Points"=w208, "Use Vertex (No)"=TRUE) -> ("Angles (deg)"=→"Angles (deg)":sgl[])  [unwired: 2 in, 2 out]
        n114 = Build Array (concatenate)(w197, w198) -> (w183:dbl[])
        "start_point_x" <- w183
        n115 = Add(x=w47, y=w46) -> (x+y=w45:dbl)
        n116 = Build Array (concatenate)(w195, w196) -> (w182:dbl[])
        "start_point_y" <- w182
        n117 = Build Array (concatenate)(w164, w193) -> (w172:dbl[])
        "end_point_y" <- w172
        n118 = Add(x=w40, y=w39) -> (x+y=w38:dbl)
        n119 = Build Array (concatenate) "创建数组"(w168, w194) -> (w176:dbl[])
        "end_point_x" <- w176
        n120 = call "IMAQ Overlay Multiple Lines 2"("Image"=w114, "Drawing Mode (Frame)"=w118, "Color"=u32 12255487, "Width"=u32 5) -> ("Image Out"=→"仅尖端轨迹":T4)  [unwired: 10 in, 1 out]
        n121 = Bundle By Name(cluster="簇 11", "next_state_x"=w45, "next_state_y"=w38, "current_state_x"=w49, "current_state_y"=w42) -> (w53:T1)
        n122 = case shown="假" "打开仅尖端轨迹" {
          tunnel: [_ w268] -> w116
          tunnel: w111 -> [_ w268]
          frame False {
          }
          frame True {
          }
        }
        n123 = Flatten To JSON(anything=w53) -> (JSON string=w57:string)  [unwired: 2 in, 1 out]
        n124 = call <vilib>:"zmq_send.vi"("data"=w57, "socket in"=w56) -> ("socket out"=w60:refnum<class "zmq_socket.lvclass">)  [unwired: 5 in, 1 out]
        n125 = call <vilib>:"zmq_recv.vi"("socket in"=w60) -> ("data"=w61:string)  [unwired: 4 in, 4 out]
        n126 = case shown="真" "打开轨迹" {
          tunnel: [_ w269] -> w213
          tunnel: w113 -> [_ w269]
          frame False {
          }
          frame True {
          }
        }
        n127 = Array Size(array=w176) -> (size(s)=w178:i32)
        n128 = call "IMAQ Overlay Multiple Lines 2"("Image"=w114, "Line End Points"=w113, "Drawing Mode (Frame)"=w125, "Color"=u32 3071, "Width"=u32 5) -> ("Image Out"=→"中心轨迹和尖端轨迹":T4)  [unwired: 9 in, 1 out]
        n129 = Unflatten From JSON "从JSON还原"(JSON string=w61, type and defaults="簇 10") -> (value=w58:T2)  [unwired: 5 in, 1 out]
        n130 = Array Size(array=w172) -> (size(s)=w174:i32)
        n131 = Subtract(x=w178, y=1) -> (x-y=w177:i32)
        n132 = Subtract(x=w174, y=1) -> (x-y=w173:i32)
        n133 = Index Array "索引数组"(array=w176, index=w177) -> (element=w163:dbl)
        "now_end_point_x" <- w163
        n134 = Subtract "delta_x"(x=w163, y=w162) -> (x-y=w134:dbl)
        "delta_x" <- w134
        n135 = Build Array (concatenate) "delta_x"(w155, w134) -> (w153:dbl[])
        n136 = Square(x=w134) -> (x^2=w159:dbl)
        n137 = Index Array "索引数组"(array=w172, index=w173) -> (element=w160:dbl)
        "now_end_point_y" <- w160
        n138 = Subtract "delta_y"(x=w160, y=w161) -> (x-y=w133:dbl)
        "delta_y" <- w133
        n139 = Build Array (concatenate) "delta_y"(w154, w133) -> (w152:dbl[])
        n140 = Square(x=w133) -> (x^2=w158:dbl)
        n141 = Add(x=w159, y=w158) -> (x+y=w157:dbl)
        n142 = Square Root(x=w157) -> (sqrt(x)=w156:dbl)
        "delta_distance" <- w156
        n143 = Divide(x=w134, y=w133) -> (x/y=w132:dbl)
        "tan(v)" <- w132
        n144 = Divide(x=w156, y=w138) -> (x/y=w137:dbl)
        "delta_velocity" <- w137
        n145 = Build Array (concatenate)(w131, w132) -> (w130:dbl[])
        n146 = Build Array (concatenate) "delta_velocity"(w136, w137) -> (w135:dbl[])
        n147 = Unbundle By Name(w58) -> ("predicted_output_dr"=w55:ext, "predicted_output_pr"=w54:ext)
        "predicted_output_dr" <- w55
        "predicted_output_pr" <- w54
        "predicted_output_dr" <- w55
        "predicted_output_pr" <- w54
        n148 = case shown="\"Rotating Field\", 默认" "Parameter Settings" {
          tunnel: w266 -> [w280 w295 w310 w329 w348 w362 w380 w395]
          tunnel: w265 -> [w277 w294 w309 w328 w346 w361 w378 w394]
          tunnel: [w279 w293 w307 w327 w347 w360 w379 w393] -> w264
          tunnel: [w278 w292 w308 w326 w345 w359 w377 w392] -> w263
          tunnel: [w273 w286 w301 w322 w339 w354 w375 w387] -> w262
          tunnel: "Pause" -> [w271 w284 w299 w321 w338 w353 w370 w385]
          tunnel: [_ _ _ w318 _ _ _ _] -> w192
          tunnel: [_ _ _ w319 _ _ _ _] -> w190
          tunnel: w110 -> [_ _ _ w317 _ _ _ _]
          tunnel: [_ _ _ w316 _ _ _ _] -> w124
          tunnel: w55 -> [_ _ _ w315 _ _ _ _]
          tunnel: w54 -> [_ _ _ w314 _ _ _ _]
          frame "Gradient Field " {
            n149 = case shown="假" w271 {
              tunnel: ["Ag" 0.0] -> w272
              frame False {
              }
              frame True {
              }
            }
            n150 = Build Array(1.0, w272, "pg", "dg", "fg") -> (w273:dbl[])
            n151 = shared-variable-write(w280, w277, w273, 1000 ("timeout ms (-1)")) -> (w279:refnum<k21>, w278:errorcluster)  [unwired: 1 out]
          }
          frame "Oscillating Field" {
            n152 = case shown="假" w284 {
              tunnel: ["AoOF" 0.0] -> w285
              frame False {
              }
              frame True {
              }
            }
            n153 = Build Array(2.0, w285, "oo", "fo", "po", "do") -> (w286:dbl[])
            n154 = shared-variable-write(w295, w294, w286, 1000 ("timeout ms (-1)")) -> (w293:refnum<k21>, w292:errorcluster)  [unwired: 1 out]
          }
          frame "Conical Field" {
            # "FG"
            n155 = case shown="假" w299 {
              tunnel: ["Ac" 0.0] -> w300
              frame False {
              }
              frame True {
              }
            }
            n156 = Build Array(3.0, w300, "wc", "pc", "dc", "cc") -> (w301:dbl[])
            n157 = shared-variable-write(w310, w309, w301, 1000 ("timeout ms (-1)")) -> (w307:refnum<k21>, w308:errorcluster)  [unwired: 1 out]
          }
          frame "Rotating Field", Default {
            n158 = case shown="假" w321 {
              tunnel: ["Ar" 0.0] -> w318
              frame False {
              }
              frame True {
              }
            }
            n159 = case shown="真" "磁场变换" {
              tunnel: [sgl 0.0 ("pr") w333] -> w324
              tunnel: [sgl 0.0 ("dr") w334] -> w319
              tunnel: w317 -> [_ w335]
              tunnel: [_ w333] -> w316
              tunnel: w315 -> [_ w334]
              tunnel: w314 -> [_ w333]
              frame False {
              }
              frame True {
                n160 = formula code="int p;\n    int q;\n    q = t/50 ;  \n    p = q%36; //用来构造循环\n    dr = -180 + (p*10);\n\n    int p2;\n    int q2;\n    q2 = q/(72);\n    p2 = q2%36; //用来构造循环\n    pr =  -40 + p2*10;"("t"=w335) -> ()  [unwired: 2 out]
                "dr" <- w334
                "pr" <- w333
              }
            }
            n161 = Build Array(4.0, w318, "wr", w324, w319) -> (w322:ext[])
            n162 = shared-variable-write "向流中写入单个元素"(w329, w328, w322, 1000 ("timeout ms (-1)")) -> (w327:refnum<k21>, w326:errorcluster)  [unwired: 1 out]
          }
          frame "Disassembly" {
            n163 = case shown="假" w338 {
              tunnel: ["Dis strength(mT)" 0.0] -> w343
              frame False {
              }
              frame True {
              }
            }
            n164 = Build Array(5.0, w343, "Dis tumbling frequency (Hz)", "Dis phase frequency (Hz)", "Dis phase step") -> (w339:dbl[])
            n165 = shared-variable-write(w348, w346, w339, 1000 ("timeout ms (-1)")) -> (w347:refnum<k21>, w345:errorcluster)  [unwired: 1 out]
          }
          frame "Swarm" {
            n166 = case shown="假" w353 {
              tunnel: ["Swa strength (mT)" 0.0] -> w352
              frame False {
              }
              frame True {
              }
            }
            n167 = Build Array(6.0, w352, "Swa frequency (Hz)", "Swa pitch angle (deg)", "Swa direction angle (deg)", "Swa ratio") -> (w354:dbl[])
            n168 = shared-variable-write(w362, w361, w354, 1000 ("timeout ms (-1)")) -> (w360:refnum<k21>, w359:errorcluster)  [unwired: 1 out]
          }
          frame "Ribbon Oscillating Field" {
            n169 = case shown="假" w370 {
              tunnel: ["Strength (mT)" 0.0] -> w369
              frame False {
              }
              frame True {
              }
            }
            n170 = Build Array(7.0, w369, "Frequency (Hz)", "Ratio (A/C)", "Direction Angle (deg)", "Pitch Angle (rotating around Origin, deg)", "Pitch Angle (rotating around Constant, deg)") -> (w375:dbl[])
            n171 = shared-variable-write(w380, w378, w375, 1000 ("timeout ms (-1)")) -> (w379:refnum<k21>, w377:errorcluster)  [unwired: 1 out]
          }
          frame "Elliptical Field" {
            n172 = case shown="假" w385 {
              tunnel: ["Ar 2" 0.0] -> w386
              frame False {
              }
              frame True {
              }
            }
            n173 = Build Array(8.0, w386, "wr  2", "pr  2", "dr  2", "ratio", "p_x") -> (w387:dbl[])
            n174 = shared-variable-write(w395, w394, w387, 1000 ("timeout ms (-1)")) -> (w393:refnum<k21>, w392:errorcluster)  [unwired: 1 out]
          }
        }
        "Array" <- w262
        "场强" <- w192
        "dr" <- w190
        n175 = Build Array (concatenate)(w189, w190) -> (w186:ext[])
        "direction angle" <- w186
        n176 = Build Array (concatenate)(w123, w124) -> (w122:ext[])
        n177 = Build Array (concatenate)(w191, w192) -> (w187:dbl[])
        "strength" <- w187
        n178 = Or(x=w263, y="Stop") -> (x .or. y?=w259:bool)
        n179 = Build Array(w188, w187, w186, w185, w180, w184, w183, w182, w176, w172, w153, w152, w139, w135, w130, w122) -> (→"all parameters":ext[][])
        "Numeric 5" <- w110
        "T" <- w110
        "T" <- w110
        "prev_end_point_x" <- w168
        "prev_end_point_y" <- w164
        "prev time" <- w147
      }
    }
    frame #3 {
      # "4. The error -314220 indicates that the other endpoint has been destroyed. The VI ignores this error."
      # "3. Destroy the stream endpoint when you click Stop or when an error occurs."
      # "Close"
      n180 = Flush Stream(8:w405, 11:w408) -> (0:w406:errorcluster, 3:w407:refnum<k21>)  [unwired: 2 in, 1 out]
      n181 = Destroy Stream Endpoint(8:w406, 11:w407) -> (0:w400:errorcluster)
      n182 = Unbundle By Name(w400) -> ("code"=w404:i32)
      n183 = xnode "Error Ring"() -> ("错误输出"=w401:errorcluster)
      n184 = Not Equal?(x=w404, y=-314220) -> (x != y?=w402:bool)
      n185 = Select(t=w400, s=w402, f=w401) -> (s? t:f=→"error out":errorcluster)
    }
  }
